vi "WaitForNotification.vi"(7 "timeout in ms (-1)":i32=-1, 8 "error in (no error)":errorcluster, 11 "Notifier in":refnum<notifier>) -> (0 "error out":errorcluster, 2 "Status out":string, 3 "Notifier out":refnum<notifier>)   [LabVIEW 2017, in "Shared Variables CD 2.0 Engine.lvlib"]
uses:
  <vilib>/Utility/error.llb/Error Cluster From Error Code.vi
  <vilib>/ErrorRing/Error Ring.xnode
  Shared Variables CD 2.0 Engine.lvlib
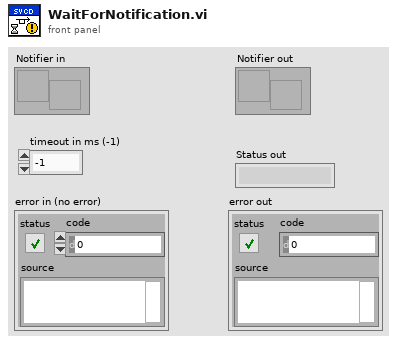
[diagram p1: front panel]
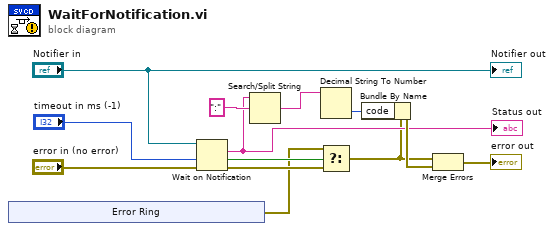
[diagram p0: block diagram]
diagram:
  n1 = xnode "Error Ring"() -> ("error out"=w3:errorcluster)
  n2 = Wait on Notification(notifier="Notifier in", timeout in ms (-1)="timeout in ms (-1)", error in (no error)="error in (no error)") -> (notification=w9:string, timed out?=w4:bool, error out=w5:errorcluster)  [unwired: 1 in, 1 out]
  "Status out" <- w9
  n3 = Search/Split String(string=w9, search string/char (-)=":") -> (match + rest of string=w11:string)  [unwired: 1 in, 2 out]
  n4 = Decimal String To Number(string=w11) -> (number=w12:i32)  [unwired: 2 in, 1 out]
  n5 = Select(t=w3, s=w4, f=w5) -> (s? t:f=w1:errorcluster)
  n6 = Bundle By Name(cluster=w1, "code"=w12) -> (w13:errorcluster)
  n7 = Merge Errors(w1, w13) -> (→"error out":errorcluster)
  "Notifier out" <- "Notifier in"
